vi "scanner cmds.vi"(8 "error in (no error)":errorcluster, 9 "data IN":string, 10 "Scanner Comands":string(combo), 11 "TCP Network Connection in":refnum<k5>) -> (0 "error out":errorcluster, 1 "CMD STAT":bool, 2 "data out":string, 3 "TCP Network Connection out":refnum<k5>, 4 "LEVEL":string, 5 "FULL BUFFER":string, 6 "BANK":string)   [LabVIEW 2017]
panel:
  in  "STA PORT CP":u16=5553
  in  "STA IP CP":string="192.168.1.53"
  out "ERROR DISPLAY":string(combo)
  out "CMD SEND":string
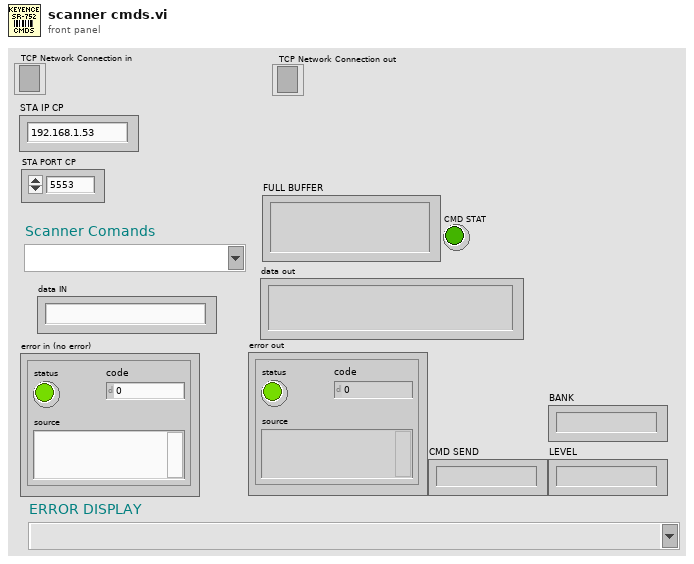
[diagram p1: front panel]
types:
  T1 = enum16{"Standard", "Buffered", "CRLF", "Immediate"}
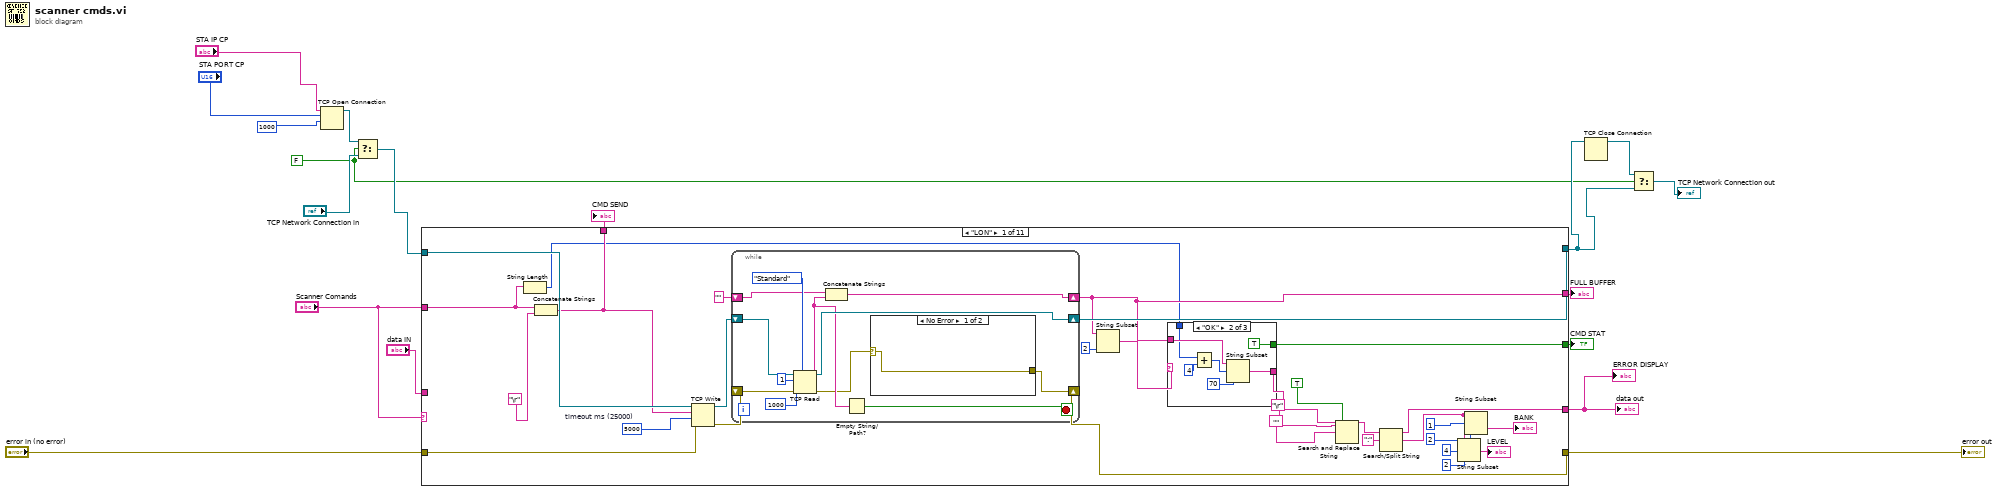
[diagram p0: block diagram]
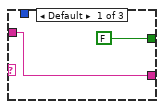
[diagram p2: hidden frame]
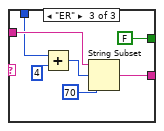
[diagram p3: hidden frame]
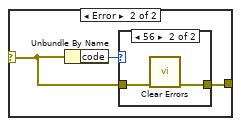
[diagram p4: hidden frame]
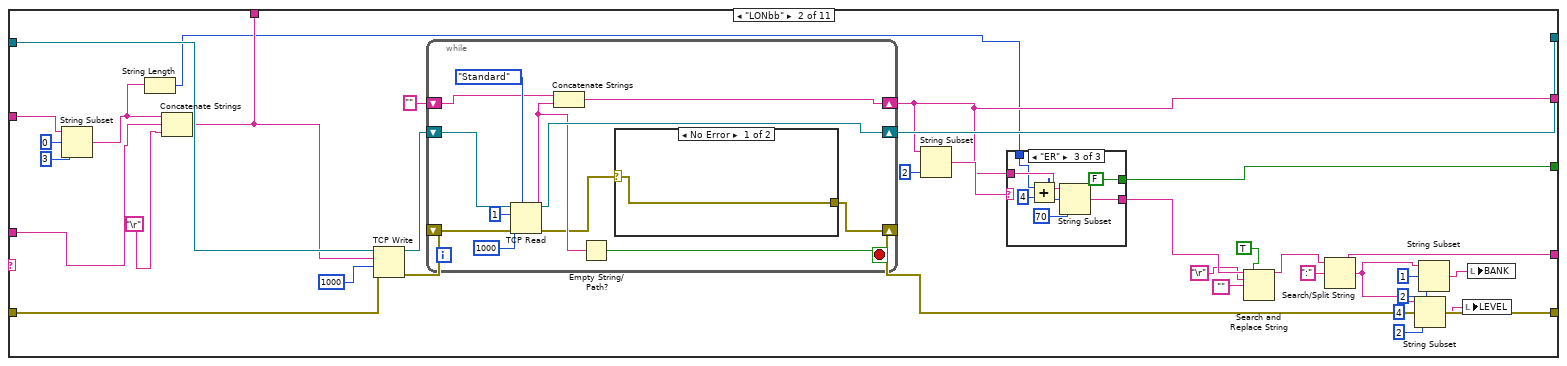
[diagram p6: hidden frame]
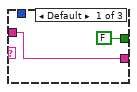
[diagram p7: hidden frame]
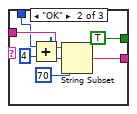
[diagram p8: hidden frame]
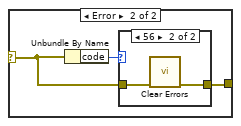
[diagram p9: hidden frame]
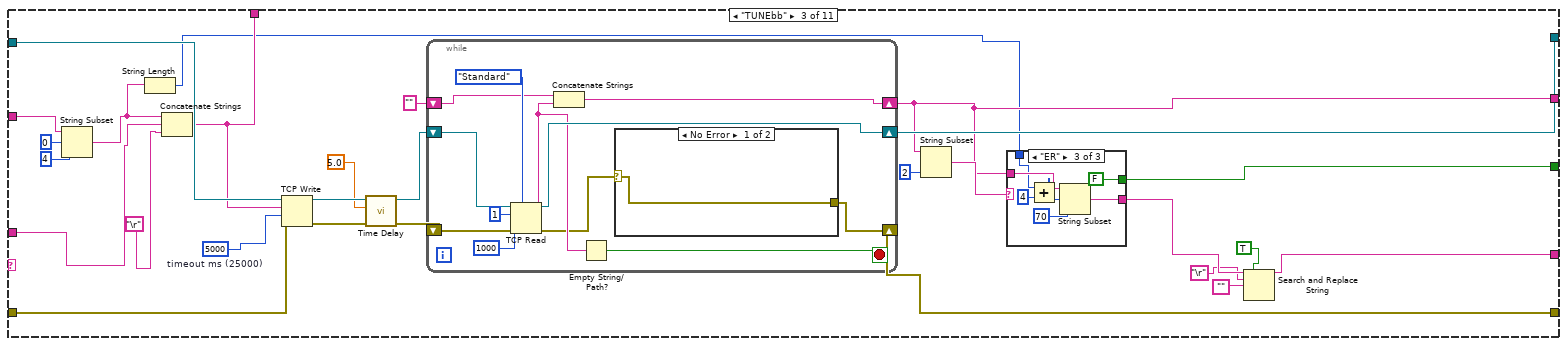
[diagram p11: hidden frame]
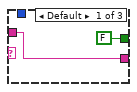
[diagram p12: hidden frame]
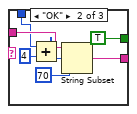
[diagram p13: hidden frame]
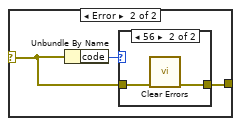
[diagram p14: hidden frame]
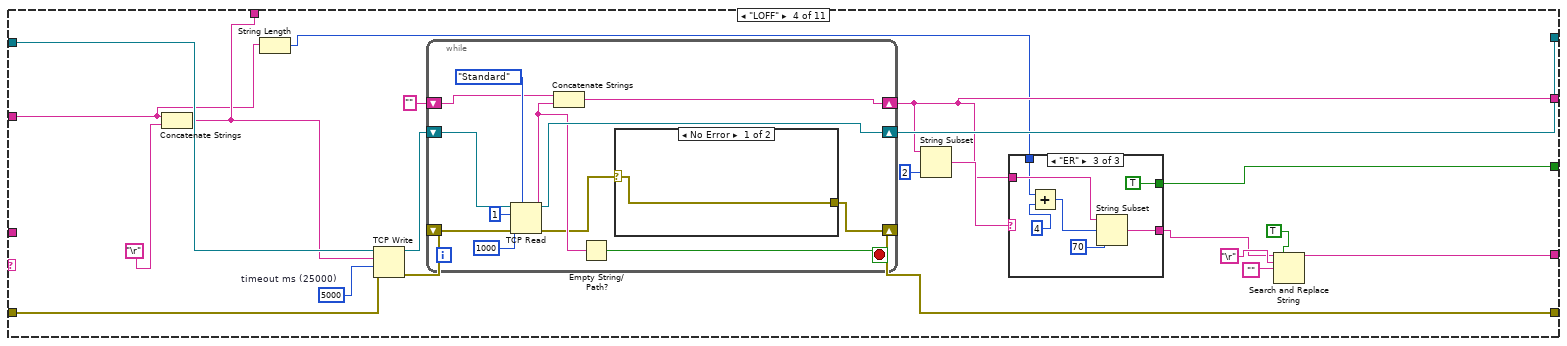
[diagram p16: hidden frame]
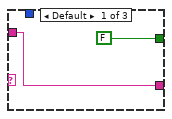
[diagram p17: hidden frame]
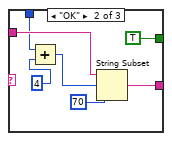
[diagram p18: hidden frame]
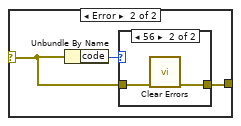
[diagram p19: hidden frame]
diagram:
  w6 = FALSE ("s")
  n1 = TCP Open Connection(address="STA IP CP", remote port or service name="STA PORT CP", timeout ms (60000)=1000 ("TCP Timeout")) -> (connection ID=w13:refnum<k5>)  [unwired: 2 in, 1 out]
  n2 = Select(t=w13, s=w6, f="TCP Network Connection in") -> (s? t:f=w14:refnum<k5>)
  n3 = case shown="\"LON\"" "Scanner Comands" {
    tunnel: "Scanner Comands" -> [w31 w100 w161 w221 w277 w335 w393 w451 w509 w567 _]
    tunnel: [w27 w89 w168 w216 w272 w330 w388 w446 w504 w563 "" ("data out")] -> w1
    tunnel: [w48 w117 w179 w235 w291 w349 w407 w465 w523 w581 w622] -> w8
    tunnel: w14 -> [w46 w115 w177 w233 w289 w347 w405 w463 w521 w579 w622]
    tunnel: [w45 w114 w176 w232 w288 w346 w404 w462 w520 w578 w624] -> w18
    tunnel: "error in (no error)" -> [w44 w113 w175 w231 w287 w345 w403 w461 w519 w577 w624]
    tunnel: [w38 w108 w170 w225 w281 w339 w397 w455 w513 w571 FALSE] -> w5
    tunnel: [w37 w107 w169 w224 w280 w338 w396 w454 w512 w570 ""] -> w4
    tunnel: [w32 w98 w159 w223 w279 w337 w395 w453 w511 w569 ""] -> w3
    tunnel: "data IN" -> [_ w97 w158 _ _ _ _ _ _ _ _]
    frame "LON" {
      w19 = 5000  # timeout ms (25000)
      n4 = String Length(string=w31) -> (length=w30:i32)
      n5 = Concatenate Strings(w31, "\r") -> (w32:string)
      n6 = TCP Write(connection ID=w46, data in=w32, error in (no error)=w44, 9:w19) -> (connection ID out=w47:refnum<k5>, error out=w43:errorcluster)  [unwired: 1 out]
      n7 = while {
        shift-right: [w76] -> w48
        shift-left: w47 -> [w75]
        shift-right: [w65] -> w45
        shift-left: w43 -> [w74]
        shift-right: [w70] -> w37
        shift-left: "" -> [w69]
        stop <- w68 stop-if-true
        n8 = TCP Read(connection ID=w75, bytes to read=1, error in (no error)=w74, 7:T1."Standard" ("mode (standard)"), 9:1000 ("timeout ms (25000)")) -> (connection ID out=w76:refnum<k5>, data out=w67:string, error out=w66:errorcluster)
        n9 = Concatenate Strings(w69, w67) -> (w70:string)
        n10 = Empty String/Path?(string/path=w67) -> (empty?=w68:bool)
        n11 = case shown="No Error" w66 {
          selector: w66 -> [w77 w78]
          tunnel: [w77 w79] -> w65
          frame No Error {
          }
          frame Error {
            n12 = Unbundle By Name(w78) -> ("code"=w80:i32)
            n13 = case shown="56" w80 {
              tunnel: [w81 w82] -> w79
              tunnel: w78 -> [w81 w83]
              frame Default {
              }
              frame 56 {
                n14 = call <vilib>:"Clear Errors.vi"("error in (no error)"=w83) -> ("error out"=w82:errorcluster)  [unwired: 5 in, 1 out]
              }
            }
          }
        }
      }
      n15 = String Subset(string=w37, length (rest)=2 ("length (rest)")) -> (substring=w39:string)  [unwired: 1 in]
      n16 = case shown="\"OK\"" w39 {
        tunnel: w37 -> [w49 w57 w64]
        tunnel: [w49 w55 w62] -> w36
        tunnel: [FALSE TRUE FALSE] -> w38
        tunnel: w30 -> [_ w53 w60]
        frame Default {
        }
        frame "OK" {
          n17 = Add(x=w53, y=4 ("offset (0)")) -> (x+y=w52:i32)
          n18 = String Subset(string=w57, offset (0)=w52, length (rest)=70 ("length (rest)")) -> (substring=w55:string)
        }
        frame "ER" {
          n19 = Add(x=w60, y=4 ("offset (0)")) -> (x+y=w59:i32)
          n20 = String Subset(string=w64, offset (0)=w59, length (rest)=70 ("length (rest)")) -> (substring=w62:string)
        }
      }
      n21 = Search and Replace String(replace all?=TRUE ("replace all? (F)"), input string=w36, search string="\r", replace string="") -> (result string=w28:string)  [unwired: 4 in, 3 out]
      n22 = Search/Split String(string=w28, search string/char (-)=":") -> (substring before match=w27:string, match + rest of string=w22:string)  [unwired: 1 in, 1 out]
      n23 = String Subset(string=w22, offset (0)=4, length (rest)=2 ("length (rest)")) -> (substring=→"LEVEL":string)
      n24 = String Subset(string=w22, offset (0)=1, length (rest)=2 ("length (rest)")) -> (substring=→"BANK":string)
    }
    frame "LONbb" {
      n25 = String Subset(string=w100, offset (0)=0, length (rest)=3 ("length (rest)")) -> (substring=w96:string)
      n26 = String Length(string=w96) -> (length=w95:i32)
      n27 = Concatenate Strings(w96, w97, "\r") -> (w98:string)
      n28 = TCP Write(connection ID=w115, data in=w98, error in (no error)=w113, 9:1000 ("TCP Timeout")) -> (connection ID out=w116:refnum<k5>, error out=w112:errorcluster)  [unwired: 1 out]
      n29 = while {
        shift-right: [w145] -> w117
        shift-left: w116 -> [w144]
        shift-right: [w134] -> w114
        shift-left: w112 -> [w143]
        shift-right: [w139] -> w107
        shift-left: "" -> [w138]
        stop <- w137 stop-if-true
        n30 = TCP Read(connection ID=w144, bytes to read=1, error in (no error)=w143, 7:T1."Standard" ("mode (standard)"), 9:1000 ("timeout ms (25000)")) -> (connection ID out=w145:refnum<k5>, data out=w136:string, error out=w135:errorcluster)
        n31 = Concatenate Strings(w138, w136) -> (w139:string)
        n32 = Empty String/Path?(string/path=w136) -> (empty?=w137:bool)
        n33 = case shown="No Error" w135 {
          selector: w135 -> [w146 w147]
          tunnel: [w146 w148] -> w134
          frame No Error {
          }
          frame Error {
            n34 = Unbundle By Name(w147) -> ("code"=w149:i32)
            n35 = case shown="56" w149 {
              tunnel: [w150 w151] -> w148
              tunnel: w147 -> [w150 w152]
              frame Default {
              }
              frame 56 {
                n36 = call <vilib>:"Clear Errors.vi"("error in (no error)"=w152) -> ("error out"=w151:errorcluster)  [unwired: 5 in, 1 out]
              }
            }
          }
        }
      }
      n37 = String Subset(string=w107, length (rest)=2 ("length (rest)")) -> (substring=w109:string)  [unwired: 1 in]
      n38 = case shown="\"ER\"" w109 {
        tunnel: w107 -> [w118 w126 w133]
        tunnel: [w118 w124 w131] -> w106
        tunnel: [FALSE TRUE FALSE] -> w108
        tunnel: w95 -> [_ w120 w127]
        frame Default {
        }
        frame "OK" {
          n39 = Add(x=w120, y=4 ("offset (0)")) -> (x+y=w121:i32)
          n40 = String Subset(string=w126, offset (0)=w121, length (rest)=70 ("length (rest)")) -> (substring=w124:string)
        }
        frame "ER" {
          n41 = Add(x=w127, y=4 ("offset (0)")) -> (x+y=w128:i32)
          n42 = String Subset(string=w133, offset (0)=w128, length (rest)=70 ("length (rest)")) -> (substring=w131:string)
        }
      }
      n43 = Search and Replace String(replace all?=TRUE ("replace all? (F)"), input string=w106, search string="\r", replace string="") -> (result string=w90:string)  [unwired: 4 in, 3 out]
      n44 = Search/Split String(string=w90, search string/char (-)=":") -> (substring before match=w89:string, match + rest of string=w85:string)  [unwired: 1 in, 1 out]
      n45 = String Subset(string=w85, offset (0)=4, length (rest)=2 ("length (rest)")) -> (substring=w93:string)
      n46 = String Subset(string=w85, offset (0)=1, length (rest)=2 ("length (rest)")) -> (substring=w86:string)
      n47 = local write "LEVEL"(w93) -> ()
      n48 = local write "BANK"(w86) -> ()
    }
    frame "TUNEbb" {
      w153 = 5000  # timeout ms (25000)
      n49 = String Subset(string=w161, offset (0)=0, length (rest)=4 ("length (rest)")) -> (substring=w157:string)
      n50 = String Length(string=w157) -> (length=w156:i32)
      n51 = Concatenate Strings(w157, w158, "\r") -> (w159:string)
      n52 = TCP Write(connection ID=w177, data in=w159, error in (no error)=w175, 9:w153) -> (connection ID out=w178:refnum<k5>, error out=w174:errorcluster)  [unwired: 1 out]
      n53 = call "Time Delay"("error in (no error)"=w174, "Delay Time (s)"=5.0) -> ("error out"=w155:errorcluster)  [unwired: 9 in]
      n54 = while {
        shift-right: [w207] -> w179
        shift-left: w178 -> [w206]
        shift-right: [w196] -> w176
        shift-left: w155 -> [w205]
        shift-right: [w201] -> w169
        shift-left: "" -> [w200]
        stop <- w199 stop-if-true
        n55 = TCP Read(connection ID=w206, bytes to read=1, error in (no error)=w205, 7:T1."Standard" ("mode (standard)"), 9:1000 ("timeout ms (25000)")) -> (connection ID out=w207:refnum<k5>, data out=w198:string, error out=w197:errorcluster)
        n56 = Concatenate Strings(w200, w198) -> (w201:string)
        n57 = Empty String/Path?(string/path=w198) -> (empty?=w199:bool)
        n58 = case shown="No Error" w197 {
          selector: w197 -> [w208 w209]
          tunnel: [w208 w210] -> w196
          frame No Error {
          }
          frame Error {
            n59 = Unbundle By Name(w209) -> ("code"=w211:i32)
            n60 = case shown="56" w211 {
              tunnel: [w212 w213] -> w210
              tunnel: w209 -> [w212 w214]
              frame Default {
              }
              frame 56 {
                n61 = call <vilib>:"Clear Errors.vi"("error in (no error)"=w214) -> ("error out"=w213:errorcluster)  [unwired: 5 in, 1 out]
              }
            }
          }
        }
      }
      n62 = String Subset(string=w169, length (rest)=2 ("length (rest)")) -> (substring=w171:string)  [unwired: 1 in]
      n63 = case shown="\"ER\"" w171 {
        tunnel: w169 -> [w180 w188 w195]
        tunnel: [w180 w186 w193] -> w167
        tunnel: [FALSE TRUE FALSE] -> w170
        tunnel: w156 -> [_ w182 w189]
        frame Default {
        }
        frame "OK" {
          n64 = Add(x=w182, y=4 ("offset (0)")) -> (x+y=w183:i32)
          n65 = String Subset(string=w188, offset (0)=w183, length (rest)=70 ("length (rest)")) -> (substring=w186:string)
        }
        frame "ER" {
          n66 = Add(x=w189, y=4 ("offset (0)")) -> (x+y=w190:i32)
          n67 = String Subset(string=w195, offset (0)=w190, length (rest)=70 ("length (rest)")) -> (substring=w193:string)
        }
      }
      n68 = Search and Replace String(replace all?=TRUE ("replace all? (F)"), input string=w167, search string="\r", replace string="") -> (result string=w168:string)  [unwired: 4 in, 3 out]
    }
    frame "LOFF" {
      w215 = 5000  # timeout ms (25000)
      n69 = Concatenate Strings(w221, "\r") -> (w223:string)
      n70 = String Length(string=w221) -> (length=w222:i32)
      n71 = TCP Write(connection ID=w233, data in=w223, error in (no error)=w231, 9:w215) -> (connection ID out=w234:refnum<k5>, error out=w230:errorcluster)  [unwired: 1 out]
      n72 = while {
        shift-right: [w263] -> w235
        shift-left: w234 -> [w262]
        shift-right: [w252] -> w232
        shift-left: w230 -> [w261]
        shift-right: [w257] -> w224
        shift-left: "" -> [w256]
        stop <- w255 stop-if-true
        n73 = TCP Read(connection ID=w262, bytes to read=1, error in (no error)=w261, 7:T1."Standard" ("mode (standard)"), 9:1000 ("timeout ms (25000)")) -> (connection ID out=w263:refnum<k5>, data out=w254:string, error out=w253:errorcluster)
        n74 = Concatenate Strings(w256, w254) -> (w257:string)
        n75 = Empty String/Path?(string/path=w254) -> (empty?=w255:bool)
        n76 = case shown="No Error" w253 {
          selector: w253 -> [w264 w265]
          tunnel: [w264 w266] -> w252
          frame No Error {
          }
          frame Error {
            n77 = Unbundle By Name(w265) -> ("code"=w267:i32)
            n78 = case shown="56" w267 {
              tunnel: [w268 w269] -> w266
              tunnel: w265 -> [w268 w270]
              frame Default {
              }
              frame 56 {
                n79 = call <vilib>:"Clear Errors.vi"("error in (no error)"=w270) -> ("error out"=w269:errorcluster)  [unwired: 5 in, 1 out]
              }
            }
          }
        }
      }
      n80 = String Subset(string=w224, length (rest)=2 ("length (rest)")) -> (substring=w226:string)  [unwired: 1 in]
      n81 = case shown="\"ER\"" w226 {
        tunnel: w224 -> [w236 w244 w251]
        tunnel: [w236 w242 w249] -> w217
        tunnel: [FALSE TRUE TRUE] -> w225
        tunnel: w222 -> [_ w238 w245]
        frame Default {
        }
        frame "OK" {
          n82 = Add(x=w238, y=4 ("length (rest)")) -> (x+y=w240:i32)
          n83 = String Subset(string=w244, offset (0)=w240, length (rest)=70 ("length (rest)")) -> (substring=w242:string)
        }
        frame "ER" {
          n84 = Add(x=w245, y=4 ("length (rest)")) -> (x+y=w247:i32)
          n85 = String Subset(string=w251, offset (0)=w247, length (rest)=70 ("length (rest)")) -> (substring=w249:string)
        }
      }
      n86 = Search and Replace String(replace all?=TRUE ("replace all? (F)"), input string=w217, search string="\r", replace string="") -> (result string=w216:string)  [unwired: 4 in, 3 out]
    }
    frame "RESET" {
      w271 = 5000  # timeout ms (25000)
      # "NEED TO REOPEN CONECTION"
      n87 = Concatenate Strings(w277, "\r") -> (w279:string)
      n88 = String Length(string=w277) -> (length=w278:i32)
      n89 = TCP Write(connection ID=w289, data in=w279, error in (no error)=w287, 9:w271) -> (connection ID out=w290:refnum<k5>, error out=w286:errorcluster)  [unwired: 1 out]
      n90 = while {
        shift-right: [w319] -> w291
        shift-left: w290 -> [w318]
        shift-right: [w308] -> w288
        shift-left: w286 -> [w317]
        shift-right: [w313] -> w280
        shift-left: "" -> [w312]
        stop <- w311 stop-if-true
        n91 = TCP Read(connection ID=w318, bytes to read=1, error in (no error)=w317, 7:T1."Standard" ("mode (standard)"), 9:1000 ("timeout ms (25000)")) -> (connection ID out=w319:refnum<k5>, data out=w310:string, error out=w309:errorcluster)
        n92 = Concatenate Strings(w312, w310) -> (w313:string)
        n93 = Empty String/Path?(string/path=w310) -> (empty?=w311:bool)
        n94 = case shown="Error" w309 {
          selector: w309 -> [w320 w321]
          tunnel: [w320 w322] -> w308
          frame No Error {
          }
          frame Error {
            n95 = Unbundle By Name(w321) -> ("code"=w323:i32)
            n96 = case shown="66" w323 {
              tunnel: [w324 w325 w327] -> w322
              tunnel: w321 -> [w324 w326 w328]
              frame Default {
              }
              frame 56 {
                n97 = call <vilib>:"Clear Errors.vi"("error in (no error)"=w326) -> ("error out"=w325:errorcluster)  [unwired: 5 in, 1 out]
              }
              frame 66 {
                n98 = call <vilib>:"Clear Errors.vi"("error in (no error)"=w328) -> ("error out"=w327:errorcluster)  [unwired: 5 in, 1 out]
              }
            }
          }
        }
      }
      n99 = String Subset(string=w280, length (rest)=2 ("length (rest)")) -> (substring=w282:string)  [unwired: 1 in]
      n100 = case shown="\"ER\"" w282 {
        tunnel: w280 -> [w292 w300 w307]
        tunnel: [w292 w298 w305] -> w273
        tunnel: [FALSE TRUE TRUE] -> w281
        tunnel: w278 -> [_ w294 w301]
        frame Default {
        }
        frame "OK" {
          n101 = Add(x=w294, y=4 ("length (rest)")) -> (x+y=w296:i32)
          n102 = String Subset(string=w300, offset (0)=w296, length (rest)=70 ("length (rest)")) -> (substring=w298:string)
        }
        frame "ER" {
          n103 = Add(x=w301, y=4 ("length (rest)")) -> (x+y=w303:i32)
          n104 = String Subset(string=w307, offset (0)=w303, length (rest)=70 ("length (rest)")) -> (substring=w305:string)
        }
      }
      n105 = Search and Replace String(replace all?=TRUE ("replace all? (F)"), input string=w273, search string="\r", replace string="") -> (result string=w272:string)  [unwired: 4 in, 3 out]
    }
    frame "BCLR" {
      w329 = 5000  # timeout ms (25000)
      # "NEED TO REOPEN CONECTION"
      n106 = Concatenate Strings(w335, "\r") -> (w337:string)
      n107 = String Length(string=w335) -> (length=w336:i32)
      n108 = TCP Write(connection ID=w347, data in=w337, error in (no error)=w345, 9:w329) -> (connection ID out=w348:refnum<k5>, error out=w344:errorcluster)  [unwired: 1 out]
      n109 = while {
        shift-right: [w377] -> w349
        shift-left: w348 -> [w376]
        shift-right: [w366] -> w346
        shift-left: w344 -> [w375]
        shift-right: [w371] -> w338
        shift-left: "" -> [w370]
        stop <- w369 stop-if-true
        n110 = TCP Read(connection ID=w376, bytes to read=1, error in (no error)=w375, 7:T1."Standard" ("mode (standard)"), 9:1000 ("timeout ms (25000)")) -> (connection ID out=w377:refnum<k5>, data out=w368:string, error out=w367:errorcluster)
        n111 = Concatenate Strings(w370, w368) -> (w371:string)
        n112 = Empty String/Path?(string/path=w368) -> (empty?=w369:bool)
        n113 = case shown="Error" w367 {
          selector: w367 -> [w378 w379]
          tunnel: [w378 w380] -> w366
          frame No Error {
          }
          frame Error {
            n114 = Unbundle By Name(w379) -> ("code"=w381:i32)
            n115 = case shown="66" w381 {
              tunnel: [w382 w383 w385] -> w380
              tunnel: w379 -> [w382 w384 w386]
              frame Default {
              }
              frame 56 {
                n116 = call <vilib>:"Clear Errors.vi"("error in (no error)"=w384) -> ("error out"=w383:errorcluster)  [unwired: 5 in, 1 out]
              }
              frame 66 {
                n117 = call <vilib>:"Clear Errors.vi"("error in (no error)"=w386) -> ("error out"=w385:errorcluster)  [unwired: 5 in, 1 out]
              }
            }
          }
        }
      }
      n118 = String Subset(string=w338, length (rest)=2 ("length (rest)")) -> (substring=w340:string)  [unwired: 1 in]
      n119 = case shown="\"ER\"" w340 {
        tunnel: w338 -> [w350 w358 w365]
        tunnel: [w350 w356 w363] -> w331
        tunnel: [FALSE TRUE TRUE] -> w339
        tunnel: w336 -> [_ w352 w359]
        frame Default {
        }
        frame "OK" {
          n120 = Add(x=w352, y=4 ("length (rest)")) -> (x+y=w354:i32)
          n121 = String Subset(string=w358, offset (0)=w354, length (rest)=70 ("length (rest)")) -> (substring=w356:string)
        }
        frame "ER" {
          n122 = Add(x=w359, y=4 ("length (rest)")) -> (x+y=w361:i32)
          n123 = String Subset(string=w365, offset (0)=w361, length (rest)=70 ("length (rest)")) -> (substring=w363:string)
        }
      }
      n124 = Search and Replace String(replace all?=TRUE ("replace all? (F)"), input string=w331, search string="\r", replace string="") -> (result string=w330:string)  [unwired: 4 in, 3 out]
    }
    frame "CMDSTAT" {
      w387 = 5000  # timeout ms (25000)
      # "NEED TO REOPEN CONECTION"
      n125 = Concatenate Strings(w393, "\r") -> (w395:string)
      n126 = String Length(string=w393) -> (length=w394:i32)
      n127 = TCP Write(connection ID=w405, data in=w395, error in (no error)=w403, 9:w387) -> (connection ID out=w406:refnum<k5>, error out=w402:errorcluster)  [unwired: 1 out]
      n128 = while {
        shift-right: [w435] -> w407
        shift-left: w406 -> [w434]
        shift-right: [w424] -> w404
        shift-left: w402 -> [w433]
        shift-right: [w429] -> w396
        shift-left: "" -> [w428]
        stop <- w427 stop-if-true
        n129 = TCP Read(connection ID=w434, bytes to read=1, error in (no error)=w433, 7:T1."Standard" ("mode (standard)"), 9:1000 ("timeout ms (25000)")) -> (connection ID out=w435:refnum<k5>, data out=w426:string, error out=w425:errorcluster)
        n130 = Concatenate Strings(w428, w426) -> (w429:string)
        n131 = Empty String/Path?(string/path=w426) -> (empty?=w427:bool)
        n132 = case shown="Error" w425 {
          selector: w425 -> [w436 w437]
          tunnel: [w436 w438] -> w424
          frame No Error {
          }
          frame Error {
            n133 = Unbundle By Name(w437) -> ("code"=w439:i32)
            n134 = case shown="66" w439 {
              tunnel: [w440 w441 w443] -> w438
              tunnel: w437 -> [w440 w442 w444]
              frame Default {
              }
              frame 56 {
                n135 = call <vilib>:"Clear Errors.vi"("error in (no error)"=w442) -> ("error out"=w441:errorcluster)  [unwired: 5 in, 1 out]
              }
              frame 66 {
                n136 = call <vilib>:"Clear Errors.vi"("error in (no error)"=w444) -> ("error out"=w443:errorcluster)  [unwired: 5 in, 1 out]
              }
            }
          }
        }
      }
      n137 = String Subset(string=w396, length (rest)=2 ("length (rest)")) -> (substring=w398:string)  [unwired: 1 in]
      n138 = case shown="\"ER\"" w398 {
        tunnel: w396 -> [w408 w416 w423]
        tunnel: [w408 w414 w421] -> w389
        tunnel: [FALSE TRUE TRUE] -> w397
        tunnel: w394 -> [_ w410 w417]
        frame Default {
        }
        frame "OK" {
          n139 = Add(x=w410, y=4 ("length (rest)")) -> (x+y=w412:i32)
          n140 = String Subset(string=w416, offset (0)=w412, length (rest)=70 ("length (rest)")) -> (substring=w414:string)
        }
        frame "ER" {
          n141 = Add(x=w417, y=4 ("length (rest)")) -> (x+y=w419:i32)
          n142 = String Subset(string=w423, offset (0)=w419, length (rest)=70 ("length (rest)")) -> (substring=w421:string)
        }
      }
      n143 = Search and Replace String(replace all?=TRUE ("replace all? (F)"), input string=w389, search string="\r", replace string="") -> (result string=w388:string)  [unwired: 4 in, 3 out]
    }
    frame "ERRSTAT" {
      w445 = 5000  # timeout ms (25000)
      # "NEED TO REOPEN CONECTION"
      n144 = Concatenate Strings(w451, "\r") -> (w453:string)
      n145 = String Length(string=w451) -> (length=w452:i32)
      n146 = TCP Write(connection ID=w463, data in=w453, error in (no error)=w461, 9:w445) -> (connection ID out=w464:refnum<k5>, error out=w460:errorcluster)  [unwired: 1 out]
      n147 = while {
        shift-right: [w493] -> w465
        shift-left: w464 -> [w492]
        shift-right: [w482] -> w462
        shift-left: w460 -> [w491]
        shift-right: [w487] -> w454
        shift-left: "" -> [w486]
        stop <- w485 stop-if-true
        n148 = TCP Read(connection ID=w492, bytes to read=1, error in (no error)=w491, 7:T1."Standard" ("mode (standard)"), 9:1000 ("timeout ms (25000)")) -> (connection ID out=w493:refnum<k5>, data out=w484:string, error out=w483:errorcluster)
        n149 = Concatenate Strings(w486, w484) -> (w487:string)
        n150 = Empty String/Path?(string/path=w484) -> (empty?=w485:bool)
        n151 = case shown="Error" w483 {
          selector: w483 -> [w494 w495]
          tunnel: [w494 w496] -> w482
          frame No Error {
          }
          frame Error {
            n152 = Unbundle By Name(w495) -> ("code"=w497:i32)
            n153 = case shown="66" w497 {
              tunnel: [w498 w499 w501] -> w496
              tunnel: w495 -> [w498 w500 w502]
              frame Default {
              }
              frame 56 {
                n154 = call <vilib>:"Clear Errors.vi"("error in (no error)"=w500) -> ("error out"=w499:errorcluster)  [unwired: 5 in, 1 out]
              }
              frame 66 {
                n155 = call <vilib>:"Clear Errors.vi"("error in (no error)"=w502) -> ("error out"=w501:errorcluster)  [unwired: 5 in, 1 out]
              }
            }
          }
        }
      }
      n156 = String Subset(string=w454, length (rest)=2 ("length (rest)")) -> (substring=w456:string)  [unwired: 1 in]
      n157 = case shown="\"ER\"" w456 {
        tunnel: w454 -> [w466 w474 w481]
        tunnel: [w466 w472 w479] -> w447
        tunnel: [FALSE TRUE TRUE] -> w455
        tunnel: w452 -> [_ w468 w475]
        frame Default {
        }
        frame "OK" {
          n158 = Add(x=w468, y=4 ("length (rest)")) -> (x+y=w470:i32)
          n159 = String Subset(string=w474, offset (0)=w470, length (rest)=70 ("length (rest)")) -> (substring=w472:string)
        }
        frame "ER" {
          n160 = Add(x=w475, y=4 ("length (rest)")) -> (x+y=w477:i32)
          n161 = String Subset(string=w481, offset (0)=w477, length (rest)=70 ("length (rest)")) -> (substring=w479:string)
        }
      }
      n162 = Search and Replace String(replace all?=TRUE ("replace all? (F)"), input string=w447, search string="\r", replace string="") -> (result string=w446:string)  [unwired: 4 in, 3 out]
    }
    frame "TQUIT" {
      w503 = 5000  # timeout ms (25000)
      # "NEED TO REOPEN CONECTION"
      n163 = Concatenate Strings(w509, "\r") -> (w511:string)
      n164 = String Length(string=w509) -> (length=w510:i32)
      n165 = TCP Write(connection ID=w521, data in=w511, error in (no error)=w519, 9:w503) -> (connection ID out=w522:refnum<k5>, error out=w518:errorcluster)  [unwired: 1 out]
      n166 = while {
        shift-right: [w551] -> w523
        shift-left: w522 -> [w550]
        shift-right: [w540] -> w520
        shift-left: w518 -> [w549]
        shift-right: [w545] -> w512
        shift-left: "" -> [w544]
        stop <- w543 stop-if-true
        n167 = TCP Read(connection ID=w550, bytes to read=1, error in (no error)=w549, 7:T1."Standard" ("mode (standard)"), 9:1000 ("timeout ms (25000)")) -> (connection ID out=w551:refnum<k5>, data out=w542:string, error out=w541:errorcluster)
        n168 = Concatenate Strings(w544, w542) -> (w545:string)
        n169 = Empty String/Path?(string/path=w542) -> (empty?=w543:bool)
        n170 = case shown="Error" w541 {
          selector: w541 -> [w552 w553]
          tunnel: [w552 w554] -> w540
          frame No Error {
          }
          frame Error {
            n171 = Unbundle By Name(w553) -> ("code"=w555:i32)
            n172 = case shown="66" w555 {
              tunnel: [w556 w557 w559] -> w554
              tunnel: w553 -> [w556 w558 w560]
              frame Default {
              }
              frame 56 {
                n173 = call <vilib>:"Clear Errors.vi"("error in (no error)"=w558) -> ("error out"=w557:errorcluster)  [unwired: 5 in, 1 out]
              }
              frame 66 {
                n174 = call <vilib>:"Clear Errors.vi"("error in (no error)"=w560) -> ("error out"=w559:errorcluster)  [unwired: 5 in, 1 out]
              }
            }
          }
        }
      }
      n175 = String Subset(string=w512, length (rest)=2 ("length (rest)")) -> (substring=w514:string)  [unwired: 1 in]
      n176 = case shown="\"ER\"" w514 {
        tunnel: w512 -> [w524 w532 w539]
        tunnel: [w524 w530 w537] -> w505
        tunnel: [FALSE TRUE TRUE] -> w513
        tunnel: w510 -> [_ w526 w533]
        frame Default {
        }
        frame "OK" {
          n177 = Add(x=w526, y=4 ("length (rest)")) -> (x+y=w528:i32)
          n178 = String Subset(string=w532, offset (0)=w528, length (rest)=70 ("length (rest)")) -> (substring=w530:string)
        }
        frame "ER" {
          n179 = Add(x=w533, y=4 ("length (rest)")) -> (x+y=w535:i32)
          n180 = String Subset(string=w539, offset (0)=w535, length (rest)=70 ("length (rest)")) -> (substring=w537:string)
        }
      }
      n181 = Search and Replace String(replace all?=TRUE ("replace all? (F)"), input string=w505, search string="\r", replace string="") -> (result string=w504:string)  [unwired: 4 in, 3 out]
    }
    frame "NUM" {
      w561 = 5000  # timeout ms (25000)
      # "NEED TO REOPEN CONECTION"
      n182 = Concatenate Strings(w567, "\r") -> (w569:string)
      n183 = String Length(string=w567) -> (length=w568:i32)
      n184 = TCP Write(connection ID=w579, data in=w569, error in (no error)=w577, 9:w561) -> (connection ID out=w580:refnum<k5>, error out=w576:errorcluster)  [unwired: 1 out]
      n185 = while {
        shift-right: [w609] -> w581
        shift-left: w580 -> [w608]
        shift-right: [w598] -> w578
        shift-left: w576 -> [w607]
        shift-right: [w603] -> w570
        shift-left: "" -> [w602]
        stop <- w601 stop-if-true
        n186 = TCP Read(connection ID=w608, bytes to read=1, error in (no error)=w607, 7:T1."Standard" ("mode (standard)"), 9:1000 ("timeout ms (25000)")) -> (connection ID out=w609:refnum<k5>, data out=w600:string, error out=w599:errorcluster)
        n187 = Concatenate Strings(w602, w600) -> (w603:string)
        n188 = Empty String/Path?(string/path=w600) -> (empty?=w601:bool)
        n189 = case shown="Error" w599 {
          selector: w599 -> [w610 w611]
          tunnel: [w610 w612] -> w598
          frame No Error {
          }
          frame Error {
            n190 = Unbundle By Name(w611) -> ("code"=w613:i32)
            n191 = case shown="66" w613 {
              tunnel: [w614 w615 w617] -> w612
              tunnel: w611 -> [w614 w616 w618]
              frame Default {
              }
              frame 56 {
                n192 = call <vilib>:"Clear Errors.vi"("error in (no error)"=w616) -> ("error out"=w615:errorcluster)  [unwired: 5 in, 1 out]
              }
              frame 66 {
                n193 = call <vilib>:"Clear Errors.vi"("error in (no error)"=w618) -> ("error out"=w617:errorcluster)  [unwired: 5 in, 1 out]
              }
            }
          }
        }
      }
      n194 = String Subset(string=w570, length (rest)=2 ("length (rest)")) -> (substring=w572:string)  [unwired: 1 in]
      n195 = case shown="\"ER\"" w572 {
        tunnel: w570 -> [w582 w590 w597]
        tunnel: [w582 w588 w595] -> w564
        tunnel: [FALSE TRUE TRUE] -> w571
        tunnel: w568 -> [_ w584 w591]
        frame Default {
        }
        frame "OK" {
          n196 = Add(x=w584, y=4 ("length (rest)")) -> (x+y=w586:i32)
          n197 = String Subset(string=w590, offset (0)=w586, length (rest)=70 ("length (rest)")) -> (substring=w588:string)
        }
        frame "ER" {
          n198 = Add(x=w591, y=4 ("length (rest)")) -> (x+y=w593:i32)
          n199 = String Subset(string=w597, offset (0)=w593, length (rest)=70 ("length (rest)")) -> (substring=w595:string)
        }
      }
      n200 = Search and Replace String(replace all?=TRUE ("replace all? (F)"), input string=w564, search string="\r", replace string="") -> (result string=w563:string)  [unwired: 4 in, 3 out]
    }
    frame Default {
    }
  }
  "data out" <- w1
  "error out" <- w18
  "CMD STAT" <- w5
  "FULL BUFFER" <- w4
  "CMD SEND" <- w3
  "ERROR DISPLAY" <- w1
  n201 = TCP Close Connection(connection ID=w8) -> (connection ID out=w7:refnum<k5>)  [unwired: 2 in, 1 out]
  n202 = Select(t=w7, s=w6, f=w8) -> (s? t:f=→"TCP Network Connection out":refnum<k5>)
